vi "Pcre2CompileContextCopy8.vi"(8 "error in":errorcluster, 11 "pCompileContext":u64 format="%.0x") -> (0 "error out":errorcluster, 2 "pCopyOfCompileContext":u64 format="%.0x", 3 "pCompileContext":u64 format="%.0x")   [LabVIEW 2021, in "libpcre2-8.lvlib"]
uses:
  libpcre2-8.lvlib
  libpcre2-8-x32.dll
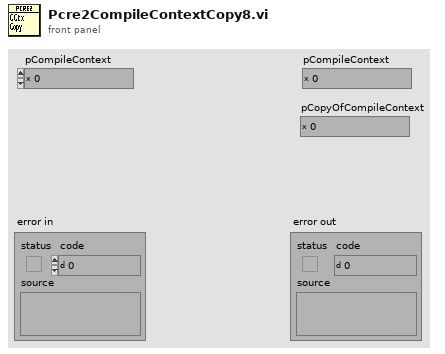
[diagram p1: front panel]
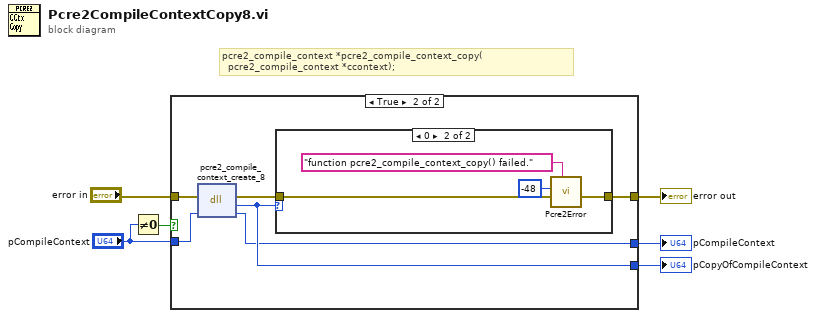
[diagram p0: block diagram]
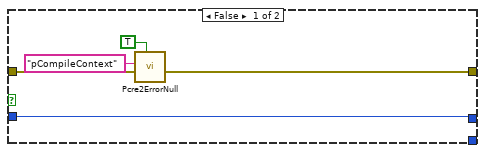
[diagram p2: hidden frame]
diagram:
  # "pcre2_compile_context *pcre2_compile_context_copy(\n  pcre2_compile_context *ccontext);"
  n1 = Not Equal To 0?(x="pCompileContext") -> (x != 0?=w1:bool)
  n2 = case shown="True" w1 {
    tunnel: "error in" -> [w10 w17]
    tunnel: [w11 w15] -> w5
    tunnel: [_ w14] -> w4
    tunnel: "pCompileContext" -> [w7 w13]
    tunnel: [w7 w12] -> w2
    frame False {
      n3 = call "Pcre2ErrorNull.vi"("IsPointer? (F)"=TRUE, "error in"=w10, "What"="pCompileContext") -> ("error out"=w11:errorcluster)  [unwired: 8 in]
    }
    frame True {
      n4 = dll-call lib="libpcre2-8-x*.dll" fn="pcre2_compile_context_create_8"(error in=w17, "ccontext"=w13) -> (error out=w16:errorcluster, "CopyOfCompileContext"=w14:u64, "ccontext"=w12:u64)  [unwired: 2 in, 1 out]
      n5 = case shown="0" w14 {
        tunnel: w16 -> [w18 w21]
        tunnel: [w18 w20] -> w15
        frame Default {
        }
        frame 0 {
          n6 = call "Pcre2Error.vi"("message"="function pcre2_compile_context_copy() failed.", "error in"=w21, "ErrorCode"=-48) -> ("error out"=w20:errorcluster)  [unwired: 8 in]
        }
      }
    }
  }
  "error out" <- w5
  "pCopyOfCompileContext" <- w4
  "pCompileContext" <- w2
